vi "SR Test Launcher.vi"() -> ()   [LabVIEW 2018]
doc: "This VI is the launcher for the Car Wash Simulator.\n\nThis VI performs any actions required to occur before the modules begin running or after they close \n(such as creating the user events). \nIt then launches the modules. The UI is launched dynamically when the program is run."
uses:
  User Events/controls/Actions.ctl
  Modules/Error Handler/Error Handler.lvlib
  Modules/Base Controller/Controller.lvlib
panel:
  out "progress":u32(slide) scale=0.0..1500.0
  in  "error in":errorcluster
  out "error out":errorcluster
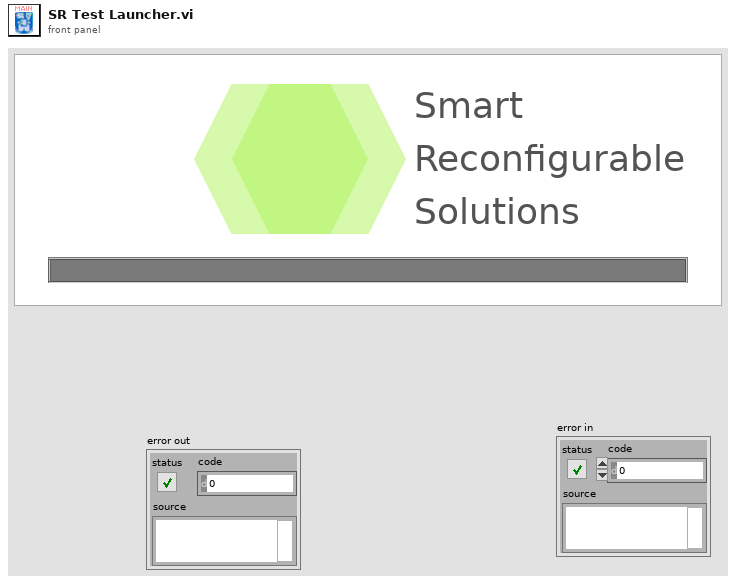
[diagram p1: front panel]
types:
  T1 = enum32{"Invalid", "Standard", "Closed", "Hidden", "Minimized", "Maximized"}
  T2 = typedef "Actions.ctl" = enum16{"Get", "Create", "Destroy"}
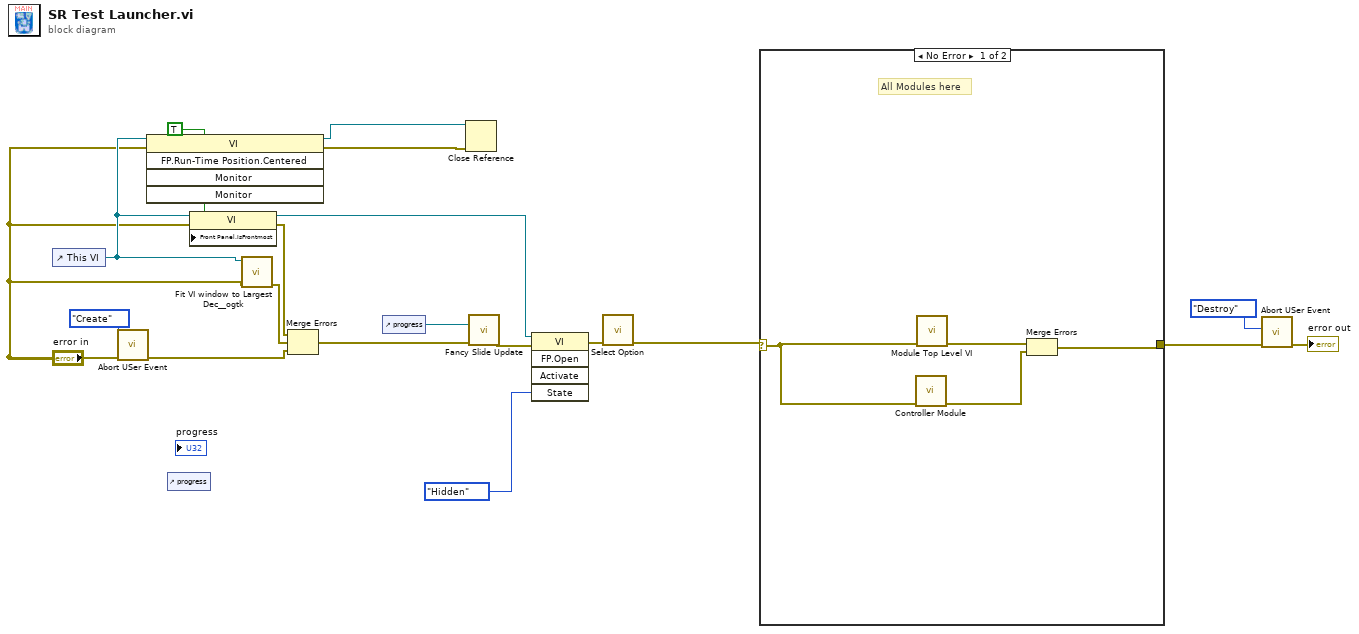
[diagram p0: block diagram]
diagram:
  n1 = control-ref of="This VI"() -> (w13:refnum<vi>)
  n2 = call "Abort USer Event.vi"("error in"="error in", "Enum"=Actions."Create") -> ("error out"=w15:errorcluster)  [unwired: 8 in, 1 out]
  n3 = invoke class="VI" method="FP.Run-Time Position.Centered"(reference=w13, error in="error in") -> (reference out=w9:refnum<vi>, error out=w5:errorcluster)  [unwired: 3 in, 3 out]
  n4 = control-ref of="progress"() -> ()  [unwired: 1 out]
  n5 = property class="VI"(reference=w13, error in="error in", "Front Panel.IsFrontmost"=TRUE ("Front Panel Window:Is Frontmost")) -> (reference out=w11:refnum<vi>, error out=w7:errorcluster)
  n6 = call <userlib>:"Fit VI window to Largest Dec__ogtk.vi"("error in (no error)"="error in", "VI Ref (calling VI)"=w13) -> ("error out"=w14:errorcluster)  [unwired: 4 in, 1 out]
  n7 = Merge Errors(w7, w14, w15) -> (w8:errorcluster)
  n8 = control-ref of="progress"() -> (w4:refnum<vi>)
  n9 = Close Reference(reference=w9, error in (no error)=w5) -> ()  [unwired: 1 out]
  n10 = call "Fancy Slide Update.vi"("error in (no error)"=w8, "Slide in"=w4) -> ("error out"=w1:errorcluster)  [unwired: 9 in]
  n11 = invoke class="VI" method="FP.Open"(reference=w11, error in=w1, "State"=T1."Hidden") -> (error out=w3:errorcluster)  [unwired: 2 in, 4 out]
  n12 = call "Select Option.vi"("error in"=w3) -> ("error out"=w2:errorcluster)  [unwired: 9 in, 1 out]
  n13 = case shown="No Error" w2 {
    selector: w2 -> [w20 w24]
    tunnel: [w22 w24] -> w18
    frame No Error {
      # "All Modules here"
      n14 = call "Controller Module.vi"("error in"=w20) -> ("error out"=w21:errorcluster)  [unwired: 10 in]
      n15 = call "Module Top Level VI.vi"("error in"=w20) -> ("error out"=w23:errorcluster)  [unwired: 10 in]
      n16 = Merge Errors(w23, w21) -> (w22:errorcluster)
    }
    frame Error {
    }
  }
  n17 = call "Abort USer Event.vi"("error in"=w18, "Enum"=Actions."Destroy") -> ("error out"=→"error out":errorcluster)  [unwired: 8 in, 1 out]
